vi "Read TestLog.vi"(11 "Model in":refnum<class "Model.lvclass">) -> (2 "ITestLog.lvclass":refnum<class "ITestLog.lvclass">, 3 "Model out":refnum<class "Model.lvclass">)   [LabVIEW 2015, in "Model.lvclass"]
uses:
  Model.lvclass
  TestLog/ITestLog/ITestLog.lvclass
  Model.lvclass/Model.ctl
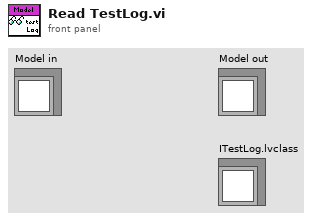
[diagram p1: front panel]
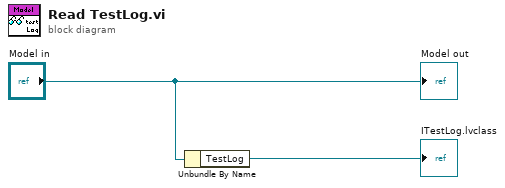
[diagram p0: block diagram]
diagram:
  n1 = Unbundle By Name("Model in") -> ("TestLog"=→"ITestLog.lvclass":refnum<class "ITestLog.lvclass">)
  "Model out" <- "Model in"
